vi "Local Transition Inward.vi"(8 "error in (no error)":errorcluster, 9 "Timeout Period in ms (-1, never)":i32=-1, 10 "Target State in":refnum<class "State Machine Actor.lvclass">, 11 "State Machine Actor in":refnum<class "State Machine Actor.lvclass">) -> (0 "error out":errorcluster, 3 "State Machine Actor out":refnum<class "State Machine Actor.lvclass">)   [LabVIEW 2024, in "State Machine Actor.lvlib" / "State Machine Actor.lvclass"]
uses:
  State Machine Actor.lvclass
  State Machine Actor.lvclass/State Machine Actor.ctl
  C:/Users/uspoaotto/OneDrive - Oregon Tool/Desktop/working copies/stateMachineActor/src/_State Machine Actor/_State Machine Actor/_State Machine Actor.lvclass
  C:/Program Files (x86)/National Instruments/LabVIEW 2024/vi.lib/ActorFramework/Actor/Actor.lvclass
  C:/Users/uspoaotto/OneDrive - Oregon Tool/Desktop/working copies/stateMachineActor/src/State Machine Actor/State Machine Actor/State Machine Actor.lvclass
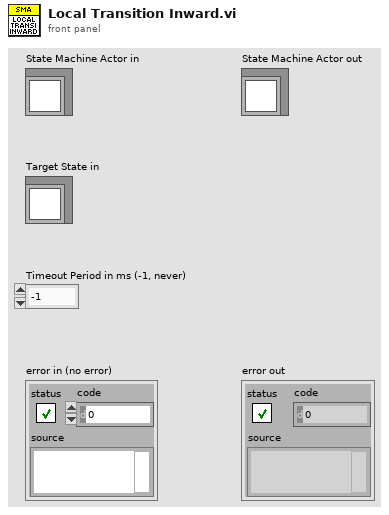
[diagram p1: front panel]
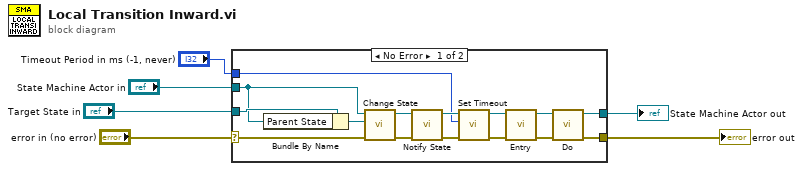
[diagram p0: block diagram]
diagram:
  n1 = case shown="No Error" "error in (no error)" {
    selector: "error in (no error)" -> [w18 w23]
    tunnel: [w9 w23] -> w5
    tunnel: "State Machine Actor in" -> [w19 w22]
    tunnel: "Timeout Period in ms (-1, never)" -> [w11 _]
    tunnel: "Target State in" -> [w21 _]
    tunnel: [w7 w22] -> w1
    frame No Error {
      n2 = Bundle By Name(cluster=w21, "Parent State"=w19) -> (w20:refnum<class "State Machine Actor.lvclass">)
      n3 = call-dynamic "Change State.vi"("error in (no error)"=w18, "Target State"=w20, "State Machine Actor in"=w19) -> ("error out"=w13:errorcluster, "State Machine Actor out"=w14:refnum<class "State Machine Actor.lvclass">)  [unwired: 7 in]
      n4 = call-dynamic "Notify State.vi"("error in (no error)"=w13, "State Machine Actor in"=w14) -> ("error out"=w16:errorcluster, "State Machine Actor out"=w12:refnum<class "State Machine Actor.lvclass">)  [unwired: 8 in]
      n5 = call-dynamic "Set Timeout.vi"("error in (no error)"=w16, "Timeout Period in ms (-1, never)"=w11, "State Machine Actor in"=w12) -> ("error out"=w15:errorcluster, "State Machine Actor out"=w10:refnum<class "State Machine Actor.lvclass">)  [unwired: 7 in]
      n6 = call-dynamic "Entry.vi"("error in (no error)"=w15, "State Machine Actor in"=w10) -> ("error out"=w17:errorcluster, "State Machine Actor out"=w8:refnum<class "State Machine Actor.lvclass">)  [unwired: 8 in]
      n7 = call-dynamic "Do.vi"("error in (no error)"=w17, "_State Machine Actor in"=w8) -> ("error out"=w9:errorcluster, "_State Machine Actor out"=w7:refnum<class "State Machine Actor.lvclass">)  [unwired: 8 in]
    }
    frame Error {
    }
  }
  "error out" <- w5
  "State Machine Actor out" <- w1
